vi "Sample SubVI 2.vi"(8 "error in (no error)":errorcluster, 11 "Numeric":u32) -> (0 "error out":errorcluster)   [LabVIEW 2019]
doc: "This VI is used to demonstrate the addition of a VI to a project."
panel:
  # "Sample SubVI 2"
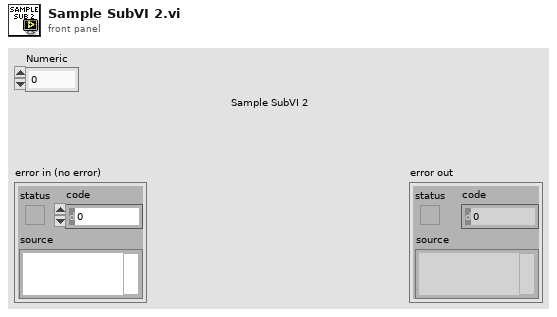
[diagram p1: front panel]
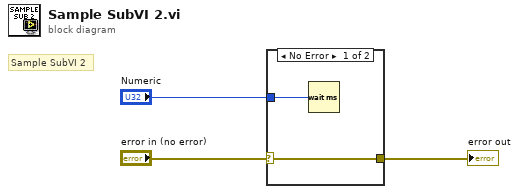
[diagram p0: block diagram]
diagram:
  # "Sample SubVI 2"
  n1 = case shown="No Error" "error in (no error)" {
    selector: "error in (no error)" -> [w5 w6]
    tunnel: [w5 w6] -> w3
    tunnel: "Numeric" -> [w4 _]
    frame No Error {
      n2 = Wait (ms)(milliseconds to wait=w4) -> ()  [unwired: 1 out]
    }
    frame Error {
    }
  }
  "error out" <- w3
